vi "Configure Routine.vi"(8 "error in (no error)":errorcluster, 9 "ID":u16=1 min=1 format="%.0x", 10 "Existing PIDs":string[](array[string]), 11 "Name":string) -> (0 "error out":errorcluster, 1 "ID out":u16, 2 "Cancel PID?":bool, 3 "Name out":string)   [LabVIEW 2015, in "Diagnostics Addon System Explorer.lvlib"]
uses:
  <vilib>/NI/AMC/Create Single Message.vi
  <vilib>/NI/AMC/Update Message Routing Info.vi
  <vilib>/NI/AMC/Read Termination Message.vi
  <vilib>/NI/AMC/Send Message.vi
  <vilib>/NI/AMC/Globals.vi
  Diagnostics Addon System Explorer.lvlib
  <vilib>/NI/AMC/AMC.lvlib
panel:
  in  "Cancel PID":bool
  in  "Apply":bool
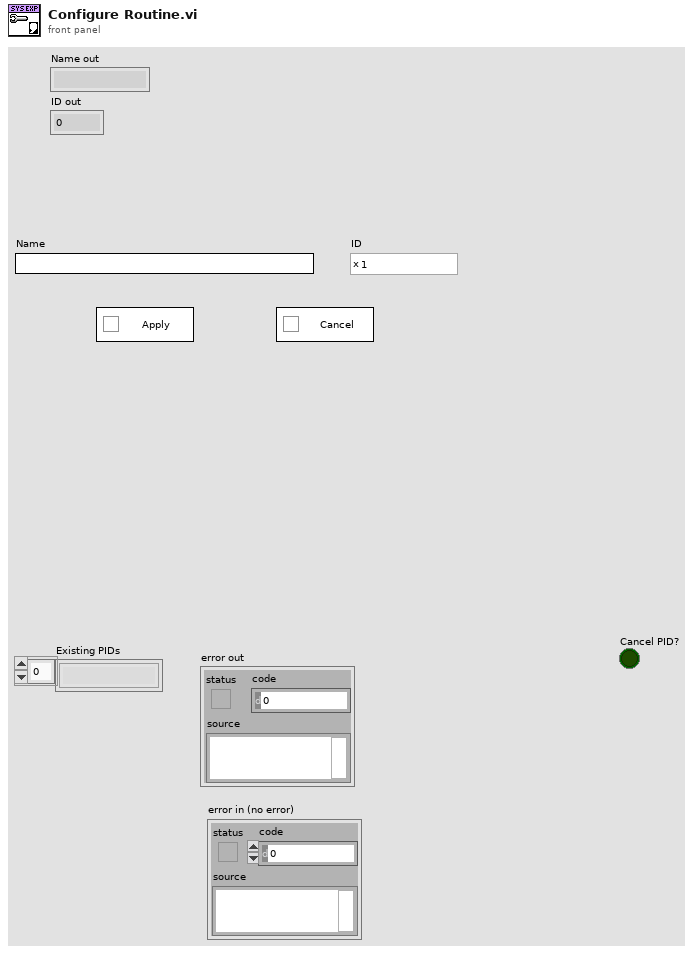
[diagram p1: front panel]
types:
  T1 = cluster{"Apply":refnum<vi>, "Cancel PID":refnum<vi>}
  T2 = typedef "AMC.lvlib/Message Queue.ctl" = refnum<queue>
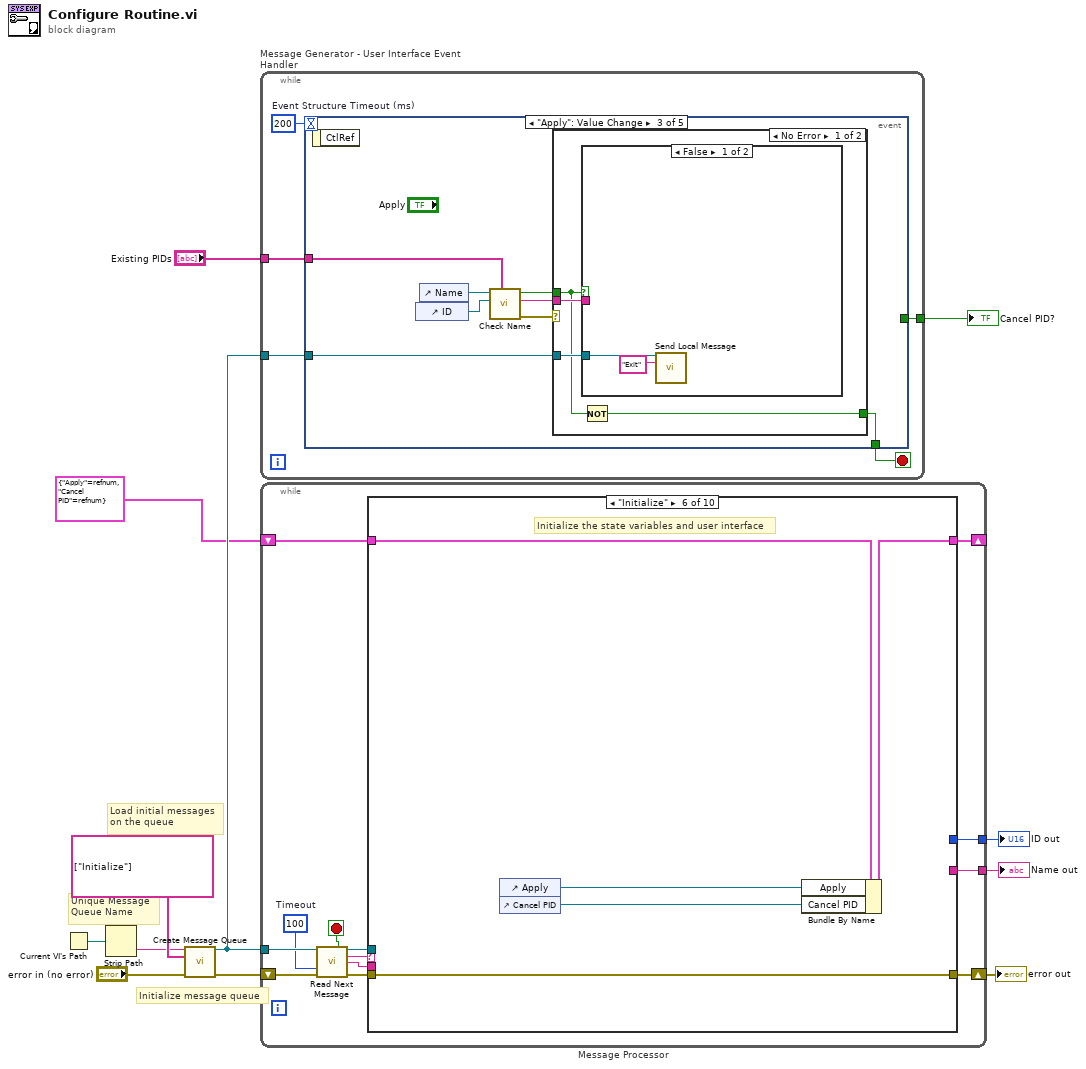
[diagram p0: block diagram]
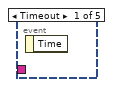
[diagram p2: hidden frame]
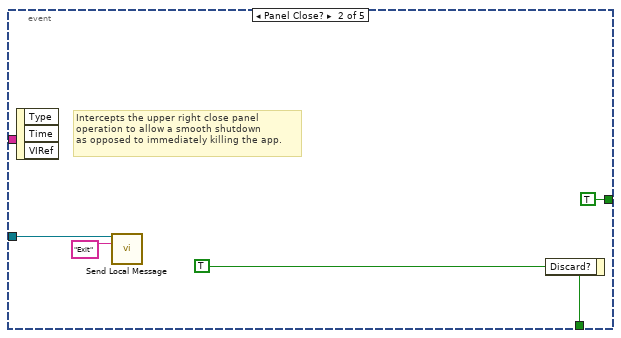
[diagram p3: hidden frame]
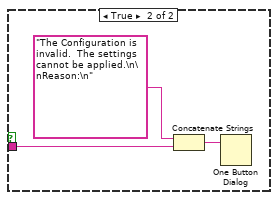
[diagram p4: hidden frame]
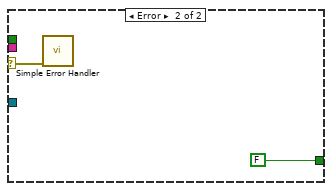
[diagram p5: hidden frame]
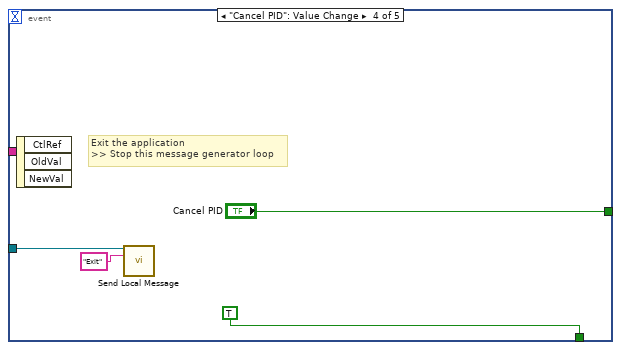
[diagram p6: hidden frame]
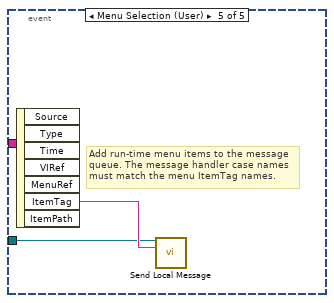
[diagram p7: hidden frame]
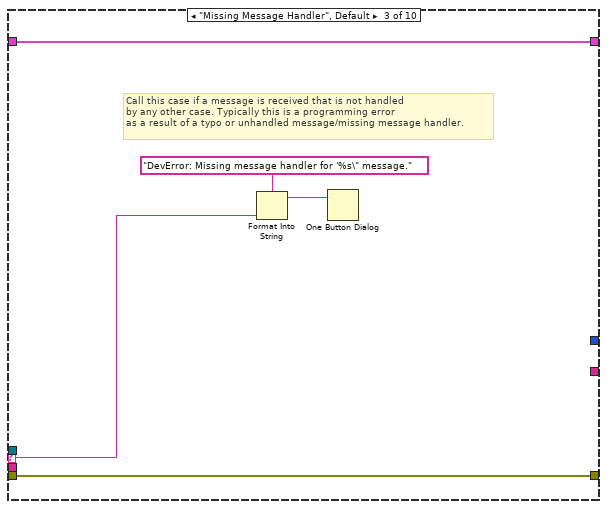
[diagram p10: hidden frame]
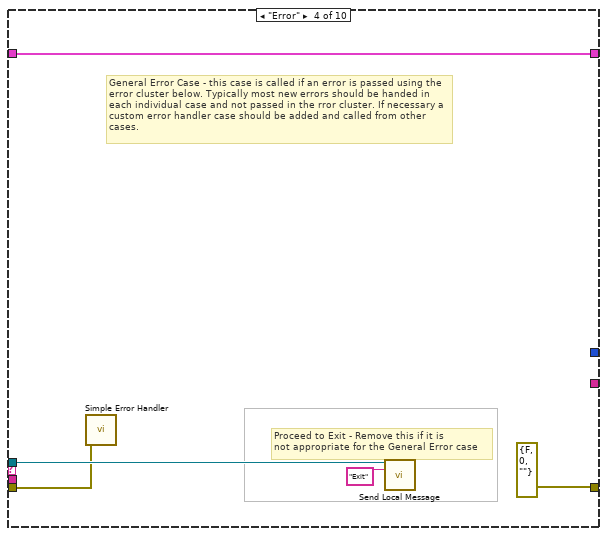
[diagram p11: hidden frame]
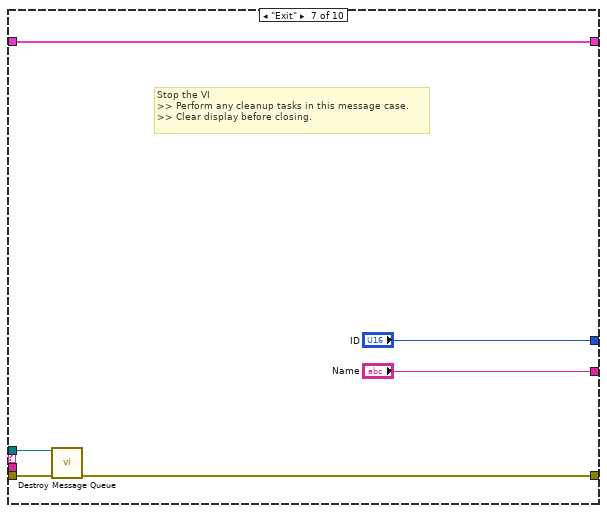
[diagram p13: hidden frame]
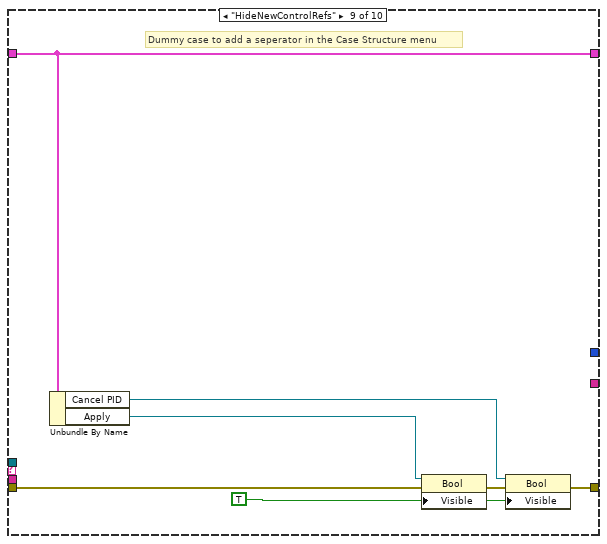
[diagram p15: hidden frame]
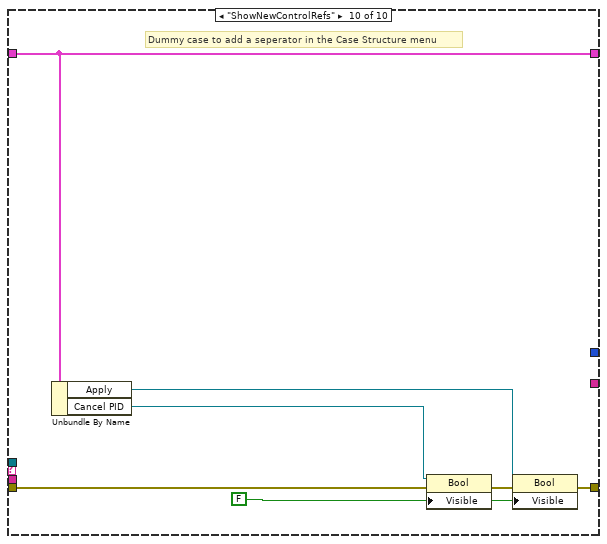
[diagram p16: hidden frame]
diagram:
  # "Initialize message queue"
  # "Unique Message\nQueue Name"
  # "Load initial messages\non the queue"
  n1 = Current VI's Path() -> (path=w8:path)
  n2 = Strip Path(path=w8) -> (name=w11:string)  [unwired: 1 out]
  n3 = call <vilib>:"Create Message Queue.vi"("message queue name"=w11, "initial message names"=string[] ["Initialize"], "error in"="error in (no error)") -> ("message queue out"=w10:T2, "error out"=w9:errorcluster)  [unwired: 11 in]
  n4 = while "Message Generator - User Interface Event Handler" {
    tunnel: w10 -> [w15]
    tunnel: [w14] -> w6
    tunnel: "Existing PIDs" -> [w13]
    stop <- w16 stop-if-true
    w17 = 200  # Event Structure Timeout (ms)
    n5 = event shown="[2] \"Apply\": Value Change" {
      selector: _ -> [_ _ _ _ _]
      dyn-events: _ -> [_ _ _ _ _]
      timeout: w17 -> [_ _ _ _ _]
      tunnel: [_ w21 w28 TRUE ("Discard?") _] -> w16
      tunnel: w15 -> [_ w19 w29 w42 w45]
      tunnel: [_ TRUE ("Cancel PID") _ "Cancel PID" _] -> w14
      tunnel: w13 -> [_ _ w22 _ _]
      event Timeout {
        n6 = event-data() -> ()  [unwired: 2 out]
      }
      event Panel Close? {
        w21 = TRUE ("Discard?")
        # "Intercepts the upper right close panel\noperation to allow a smooth shutdown\nas opposed to immediately killing the app."
        n7 = event-data() -> ()  [unwired: 4 out]
        n8 = call <vilib>:"Send Local Message.vi"("message queue in"=w19, "message name"="Exit") -> ()  [unwired: 11 in, 3 out]
        n9 = event-data("Discard?"=w21) -> ()  [unwired: 1 in, 1 out]
      }
      event "Apply": Value Change {
        n10 = event-data() -> ()  [unwired: 2 out]
        n11 = control-ref of="ID"() -> (w24:refnum<vi>)
        n12 = control-ref of="Name"() -> (w23:refnum<vi>)
        n13 = call "Check Name.vi"("Existing PIDs"=w22, "ID"=w24, "Name"=w23) -> ("error out"=w27:errorcluster, "String"=w25:string, "Boolean"=w26:bool)  [unwired: 6 in]
        n14 = case shown="No Error" w27 {
          selector: w27 -> [_ w40]
          tunnel: w26 -> [w31 _]
          tunnel: w29 -> [w33 _]
          tunnel: w25 -> [w32 _]
          tunnel: [w30 FALSE] -> w28
          frame No Error {
            n15 = case shown="False" w31 {
              tunnel: w33 -> [w35 _]
              tunnel: w32 -> [_ w38]
              frame False {
                n16 = call <vilib>:"Send Local Message.vi"("message queue in"=w35, "message name"="Exit" ("Message Name")) -> ()  [unwired: 11 in, 3 out]
              }
              frame True {
                n17 = Concatenate Strings("The Configuration is invalid.  The settings cannot be applied.\n\nReason:\n" ("message"), w38) -> (w36:string)
                n18 = One Button Dialog(message=w36) -> ()  [unwired: 1 in, 1 out]
              }
            }
            n19 = Not(x=w31) -> (.not. x?=w30:bool)
          }
          frame Error {
            n20 = call <vilib>:"Simple Error Handler.vi"("error in (no error)"=w40) -> ()  [unwired: 4 in, 5 out]
          }
        }
      }
      event "Cancel PID": Value Change {
        # "Exit the application\n>> Stop this message generator loop"
        n21 = event-data() -> ()  [unwired: 4 out]
        n22 = call <vilib>:"Send Local Message.vi"("message queue in"=w42, "message name"="Exit") -> ()  [unwired: 11 in, 3 out]
      }
      event Menu Selection (User) {
        # "Add run-time menu items to the message\nqueue. The message handler case names must match the menu ItemTag names."
        n23 = event-data() -> ("ItemTag"=w46:string)  [unwired: 7 out]
        n24 = call <vilib>:"Send Local Message.vi"("message queue in"=w45, "message name"=w46) -> ()  [unwired: 11 in, 3 out]
      }
    }
  }
  "Cancel PID?" <- w6
  n25 = while "Message Processor" {
    shift-left: w9 -> [w53]
    shift-right: [w57] -> w4
    tunnel: w10 -> [w54]
    shift-left: T1 {"Apply"=refnum, "Cancel PID"=refnum} ("State Variables") -> [w59]
    shift-right: [w58] -> _
    tunnel: [w48] -> w2
    tunnel: [w47] -> w1
    stop <- w56 stop-if-true
    w51 = 100  # Timeout
    n26 = call <vilib>:"Read Next Message.vi"("message queue in"=w54, "timeout (1 ms)"=w51, "error in"=w53) -> ("exit process?"=w56:bool, "message queue out"=w55:T2, "message name"=w50:string, "message value"=w49:string, "error out"=w52:errorcluster)  [unwired: 5 in, 3 out]
    n27 = case shown="\"Initialize\"" w50 {
      selector: w50 -> [_ _ w66 _ _ _ _ _ _ _]
      tunnel: [w61 w63 w68 w73 w75 w79 w84 w88 w95 w102] -> w58
      tunnel: w59 -> [w61 w63 w68 w73 w75 w80 w84 w88 w95 w102]
      tunnel: w55 -> [_ _ _ w71 _ _ w85 _ _ _]
      tunnel: w52 -> [w60 w62 w67 w69 w74 w78 w86 w87 w89 w96]
      tunnel: [w60 w62 w67 errorcluster {"status"=FALSE, "code"=0, "source"=""} ("error out") w74 w78 w83 w87 w92 w100] -> w57
      tunnel: w49 -> [_ _ _ _ _ _ _ _ _ _]
      tunnel: [_ _ _ _ _ _ "Name" _ _ _] -> w48
      tunnel: [_ _ _ _ _ _ "ID" _ _ _] -> w47
      frame "---------- Framework Operations ----------" {
        # "Dummy case to add a seperator in the Case Structure menu"
      }
      frame "", "Idle" {
        # "Idle Case - this case is called after a Timeout on the Get Next Message from Queue VI, if no new messages are present on the queue. This case can be used for housekeeping tasks such as updating the UI."
      }
      frame "Missing Message Handler", Default {
        # "Call this case if a message is received that is not handled \nby any other case. Typically this is a programming error\nas a result of a typo or unhandled message/missing message handler."
        n28 = Format Into String(format string="DevError: Missing message handler for '%s\" message." ("message"), w66) -> (resulting string=w64:string)  [unwired: 2 in, 1 out]
        n29 = One Button Dialog(message=w64) -> ()  [unwired: 2 out]
      }
      frame "Error" {
        # "Proceed to Exit - Remove this if it is\nnot appropriate for the General Error case"
        # "General Error Case - this case is called if an error is passed using the error cluster below. Typically most new errors should be handed in each individual case and not passed in the rror cluster. If necessary a custom error handler case should be added and called from other cases."
        n30 = call <vilib>:"Simple Error Handler.vi"("error in (no error)"=w69) -> ()  [unwired: 1 in, 8 out]
        n31 = call <vilib>:"Send Local Message.vi"("message queue in"=w71, "message name"="Exit") -> ()  [unwired: 11 in, 3 out]
      }
      frame "---------- Generic Operations ----------" {
        # "Dummy case to add a seperator in the Case Structure menu"
      }
      frame "Initialize" {
        # "Initialize the state variables and user interface"
        n32 = control-ref of="Apply"() -> (w77:refnum<vi>)
        n33 = control-ref of="Cancel PID"() -> (w76:refnum<vi>)
        n34 = Bundle By Name(cluster=w80, "Apply"=w77, "Cancel PID"=w76) -> (w79:T1)
      }
      frame "Exit" {
        # "Stop the VI\n>> Perform any cleanup tasks in this message case.\n>> Clear display before closing."
        n35 = call <vilib>:"Destroy Message Queue.vi"("message queue in"=w85, "error in"=w86) -> ("error out"=w83:errorcluster)  [unwired: 11 in, 2 out]
      }
      frame "---------- Application Operations ----------" {
        # "Dummy case to add a seperator in the Case Structure menu"
      }
      frame "HideNewControlRefs" {
        w93 = TRUE ("Visible")
        # "Dummy case to add a seperator in the Case Structure menu"
        n36 = Unbundle By Name(w95) -> ("Cancel PID"=w90:refnum<vi>, "Apply"=w91:refnum<vi>)
        n37 = property class="Bool"(reference=w91, error in=w89, "Visible"=w93) -> (error out=w94:errorcluster)  [unwired: 1 out]
        n38 = property class="Bool"(reference=w90, error in=w94, "Visible"=w93) -> (error out=w92:errorcluster)  [unwired: 1 out]
      }
      frame "ShowNewControlRefs" {
        w99 = FALSE ("Visible")
        # "Dummy case to add a seperator in the Case Structure menu"
        n39 = Unbundle By Name(w102) -> ("Apply"=w98:refnum<vi>, "Cancel PID"=w97:refnum<vi>)
        n40 = property class="Bool"(reference=w97, error in=w96, "Visible"=w99) -> (error out=w101:errorcluster)  [unwired: 1 out]
        n41 = property class="Bool"(reference=w98, error in=w101, "Visible"=w99) -> (error out=w100:errorcluster)  [unwired: 1 out]
      }
    }
  }
  "error out" <- w4
  "Name out" <- w2
  "ID out" <- w1
